vi "Initialize.vi"(8 "Error In":errorcluster, 10 "Reader":refnum<class "Reader.lvclass">, 11 "Lexer In":refnum<class "Lexer.lvclass">) -> (0 "Error Out":errorcluster, 3 "Lexer Out":refnum<class "Lexer.lvclass">)   [LabVIEW 2018, in "Toolkit.lvlib" / "Lexer.lvclass"]
doc: "Creates a new <B>Lexer</B> object.\n\n<B>Reader</B> - Represents an implementation for reading a Mustache template byte-by-byte.\n\n<B>Lexer</B> - Represents an implementation capable of identifying tokens as bytes are read from a Mustache template."
uses:
  Lexer.lvclass
  Readers/Reader/Reader.lvclass
  Lexer.lvclass/Lexer.ctl
  Type Definitions/Delimiters.ctl
  Abstract/States.ctl
  Abstract/Tag Types.ctl
  Tokens/Token/Token.lvclass
  Toolkit.lvlib
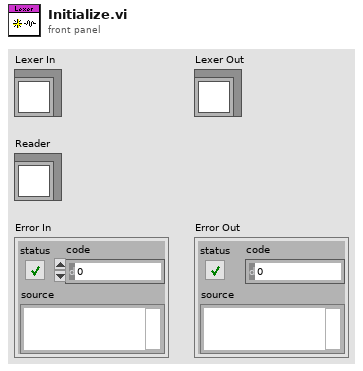
[diagram p1: front panel]
types:
  T1 = typedef "Toolkit.lvlib/Lexer.lvclass/Tag Types.ctl" = enum16{"Escaped Variable", "{} Unescaped Variable", "& Unescaped Variable", "Begin Section", "Inverted Section", "End Section", "Comment", "Partial", "Set Delimiter"}
  T2 = typedef "Toolkit.lvlib/Lexer.lvclass/States.ctl" = enum16{"Text", "Open Delimiter", "Tag Type", "Tag Key", "Close Delimiter"}
  T3 = typedef "Toolkit.lvlib/Delimiters.ctl" = cluster{"Close":string, "Open":string}
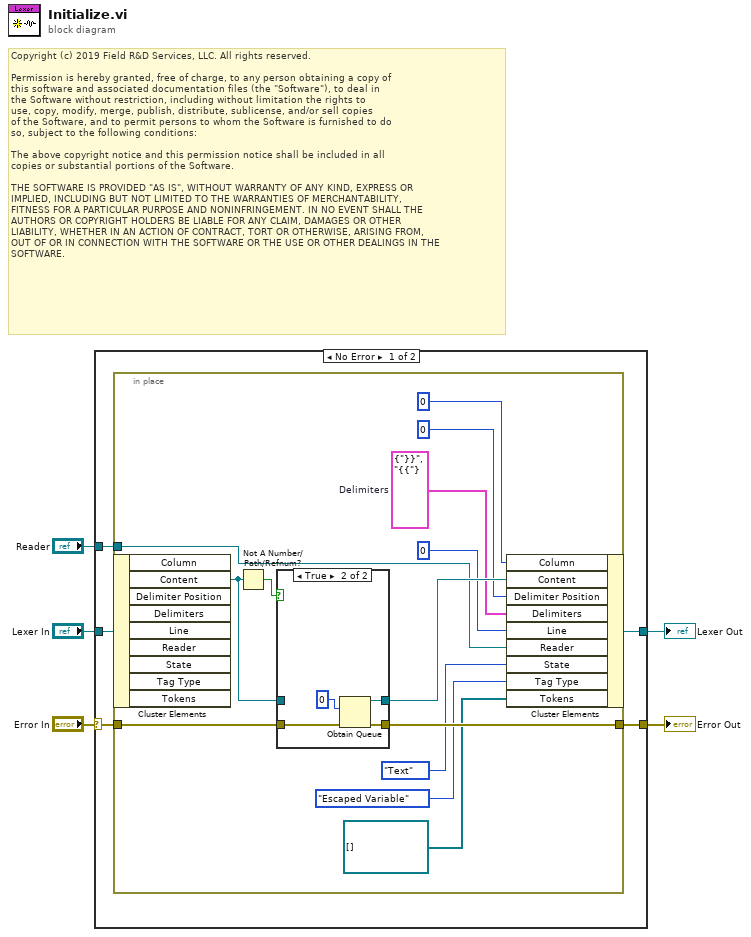
[diagram p0: block diagram]
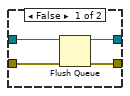
[diagram p2: hidden frame]
diagram:
  # "Copyright (c) 2019 Field R&D Services, LLC. All rights reserved.\n\nPermission is hereby granted, free of charge, to any person obtaining a copy of\nthis software and associated documentation files (the \"Software\"), to deal in\nthe Software without restriction, including without limitation the rights to\nuse, copy, modify, merge, publish, distribute, sublicense, and/or sell copies\nof the Software, and to permit persons to whom the Software is furnished to do\nso, subject to the following conditions:\n\nThe above copyright notice and this permission notice shall be included in all\ncopies or substantial portions of the Software.\n\nTHE SOFTWARE IS PROVIDED \"AS IS\", WITHOUT WARRANTY OF ANY KIND, EXPRESS OR\nIMPLIED, INCLUDING BUT NOT LIMITED TO THE WARRANTIES OF MERCHANTABILITY,\nFITNESS FOR A PARTICULAR PURPOSE AND NONINFRINGEMENT. IN NO EVENT SHALL THE\nAUTHORS OR COPYRIGHT HOLDERS BE LIABLE FOR ANY CLAIM, DAMAGES OR OTHER\nLIABILITY, WHETHER IN AN ACTION OF CONTRACT, TORT OR OTHERWISE, ARISING FROM,\nOUT OF OR IN CONNECTION WITH THE SOFTWARE OR THE USE OR OTHER DEALINGS IN THE\nSOFTWARE."
  n1 = case shown="No Error" "Error In" {
    selector: "Error In" -> [w10 w33]
    tunnel: [w9 w33] -> w4
    tunnel: "Lexer In" -> [w8 w32]
    tunnel: [w7 w32] -> w2
    tunnel: "Reader" -> [w6 _]
    frame No Error {
      n2 = in-place {
        in-place-border: w10 -> [w23]
        in-place-border: [w22] -> w9
        in-place-border: w6 -> [w11]
        w16 = T3 {"Close"="}}", "Open"="{{"}  # Delimiters
        n3 = in-place-cluster #1(w8) -> ("Content"=w20:refnum<queue>)  [unwired: 8 out]
        n4 = Not A Number/Path/Refnum?(number/path/refnum=w20) -> (NaN/Path/Refnum?=w21:bool)
        n5 = case shown="True" w21 {
          tunnel: w23 -> [w25 w31]
          tunnel: [w24 w30] -> w22
          tunnel: w20 -> [w27 _]
          tunnel: [w26 w28] -> w19
          frame False {
            n6 = Flush Queue(queue=w27, error in (no error)=w25) -> (queue out=w26:refnum<queue>, error out=w24:errorcluster)  [unwired: 1 out]
          }
          frame True {
            n7 = Obtain Queue(element data type=u8 0, error in (no error)=w31) -> (queue out=w28:refnum<queue>, error out=w30:errorcluster)  [unwired: 3 in, 1 out]
          }
        }
        n8 = in-place-cluster #1("Column"=u64 0, "Content"=w19, "Delimiter Position"=0, "Delimiters"=w16, "Line"=u64 0, "Reader"=w11, "State"=States."Text", "Tag Type"=Tag_Types."Escaped Variable", "Tokens"=refnum<class "Token.lvclass">[] []) -> (w7:refnum<class "Lexer.lvclass">)
      }
    }
    frame Error {
    }
  }
  "Error Out" <- w4
  "Lexer Out" <- w2
